vi "Drive encoders.vi"() -> (0 "encoderIzquierdoAtras":dbl, 1 "encoderDerechoAtras":dbl, 2 "encoderIzquierdoDelante":dbl, 3 "encoderDerechoDelante":dbl)   [LabVIEW 2014]
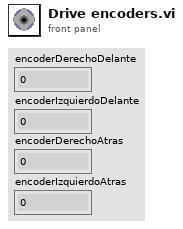
[diagram p1: front panel]
types:
  T1 = typedef "WPI_EncoderDevRef.ctl" = cluster{"DevStatus":errorcluster, "EncoderIndex":T2, "CounterIndex":T3, "DistancePerCount":dbl, "Decoding Type":T4}
  T2 = typedef "FPGA_EncoderIdx.ctl" = enum8{"Enc 0", "Enc 1", "Enc 2", "Enc 3", "Enc 4", "Enc 5", "Enc 6", "Enc 7", "Invalid"}
  T3 = typedef "FPGA_CounterCtrSystemIndex.ctl" = enum8{"Ctr 0", "Ctr 1", "Ctr 2", "Ctr 3", "Ctr 4", "Ctr 5", "Ctr 6", "Ctr 7", "Invalid"}
  T4 = typedef "WPI_EncoderType.ctl" = enum16{"1x", "2x", "4x"}
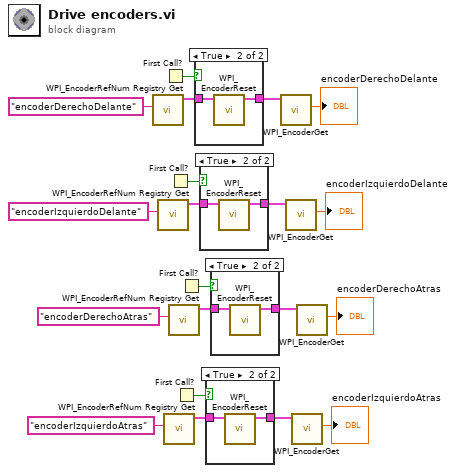
[diagram p0: block diagram]
diagram:
  n1 = call <vilib>:"WPI_EncoderRefNum Registry Get.vi"("refnum name"="encoderDerechoDelante") -> ("EncoderDevRef"=w19:T1)  [unwired: 9 in, 1 out]
  n2 = call <vilib>:"WPI_EncoderRefNum Registry Get.vi"("refnum name"="encoderIzquierdoDelante") -> ("EncoderDevRef"=w17:T1)  [unwired: 9 in, 1 out]
  n3 = First Call?() -> (First Call?: T/F=w20:bool)
  n4 = call <vilib>:"WPI_EncoderRefNum Registry Get.vi"("refnum name"="encoderIzquierdoAtras") -> ("EncoderDevRef"=w13:T1)  [unwired: 9 in, 1 out]
  n5 = First Call?() -> (First Call?: T/F=w1:bool)
  n6 = call <vilib>:"WPI_EncoderRefNum Registry Get.vi"("refnum name"="encoderDerechoAtras") -> ("EncoderDevRef"=w15:T1)  [unwired: 9 in, 1 out]
  n7 = First Call?() -> (First Call?: T/F=w3:bool)
  n8 = First Call?() -> (First Call?: T/F=w2:bool)
  n9 = case shown="True" w20 {
    tunnel: w19 -> [w21 w23]
    tunnel: [w21 w22] -> w18
    frame False {
    }
    frame True {
      n10 = call <vilib>:"WPI_EncoderReset.vi"("EncoderDevRef"=w23) -> ("EncoderDevRef"=w22:T1)  [unwired: 9 in, 1 out]
    }
  }
  n11 = case shown="True" w1 {
    tunnel: w17 -> [w24 w26]
    tunnel: [w24 w25] -> w16
    frame False {
    }
    frame True {
      n12 = call <vilib>:"WPI_EncoderReset.vi"("EncoderDevRef"=w26) -> ("EncoderDevRef"=w25:T1)  [unwired: 9 in, 1 out]
    }
  }
  n13 = case shown="True" w3 {
    tunnel: w13 -> [w27 w29]
    tunnel: [w27 w28] -> w12
    frame False {
    }
    frame True {
      n14 = call <vilib>:"WPI_EncoderReset.vi"("EncoderDevRef"=w29) -> ("EncoderDevRef"=w28:T1)  [unwired: 9 in, 1 out]
    }
  }
  n15 = case shown="True" w2 {
    tunnel: w15 -> [w30 w32]
    tunnel: [w30 w31] -> w14
    frame False {
    }
    frame True {
      n16 = call <vilib>:"WPI_EncoderReset.vi"("EncoderDevRef"=w32) -> ("EncoderDevRef"=w31:T1)  [unwired: 9 in, 1 out]
    }
  }
  n17 = call <vilib>:"WPI_EncoderGet.vi"("EncoderDevRef"=w18) -> ("Distance"=→"encoderDerechoDelante":dbl)  [unwired: 5 in, 5 out]
  n18 = call <vilib>:"WPI_EncoderGet.vi"("EncoderDevRef"=w16) -> ("Distance"=→"encoderIzquierdoDelante":dbl)  [unwired: 5 in, 5 out]
  n19 = call <vilib>:"WPI_EncoderGet.vi"("EncoderDevRef"=w12) -> ("Distance"=→"encoderIzquierdoAtras":dbl)  [unwired: 5 in, 5 out]
  n20 = call <vilib>:"WPI_EncoderGet.vi"("EncoderDevRef"=w14) -> ("Distance"=→"encoderDerechoAtras":dbl)  [unwired: 5 in, 5 out]
